vi "InjA-HMI-tester.vi"() -> ()   [LabVIEW 2016]
panel:
  out "InjectorA FPGA error":errorcluster
  out "InjectorA RT error":errorcluster
  in  "stop":bool
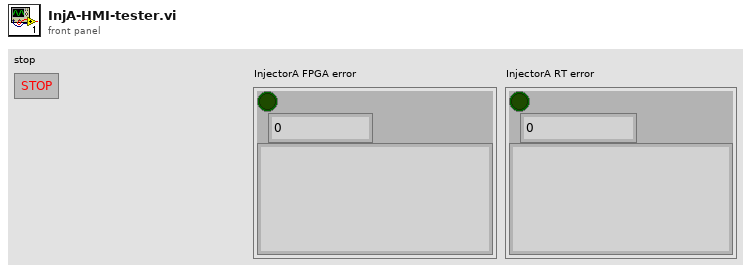
[diagram p1: front panel]
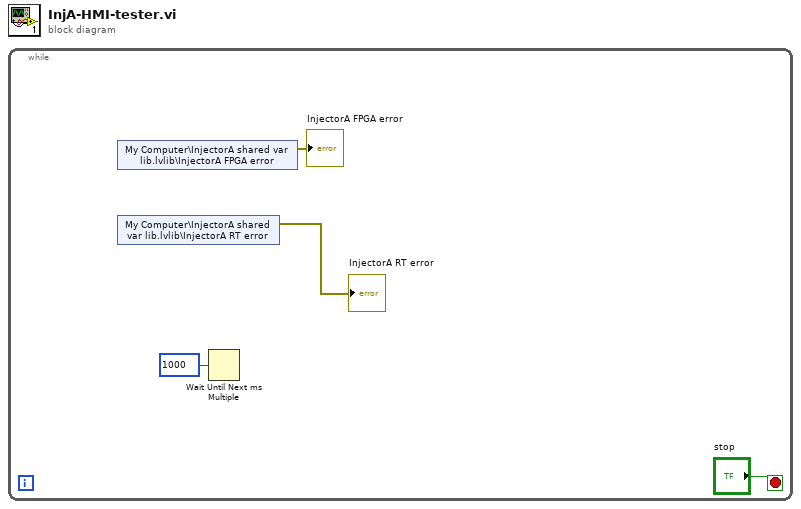
[diagram p0: block diagram]
diagram:
  n1 = while {
    stop <- "stop" stop-if-true
    n2 = shared-variable "My Computer\\InjectorA shared var lib.lvlib\\InjectorA FPGA error"() -> (→"InjectorA FPGA error":errorcluster)  [unwired: 1 in, 1 out]
    n3 = shared-variable "My Computer\\InjectorA shared var lib.lvlib\\InjectorA RT error"() -> (→"InjectorA RT error":errorcluster)  [unwired: 1 in, 1 out]
    n4 = Wait Until Next ms Multiple(millisecond multiple=u32 1000) -> ()  [unwired: 1 out]
  }
